vi "VISA Init --GPS--.vi"(2 "Error In":errorcluster, 3 "VISA resource name In":refnum<visa-resource-name>) -> (0 "Error Out":errorcluster, 1 "VISA resource name Out":refnum<visa-resource-name>)   [LabVIEW 2015]
uses:
  <vilib>/Instr/_visa.llb/VISA Configure Serial Port (Instr).vi
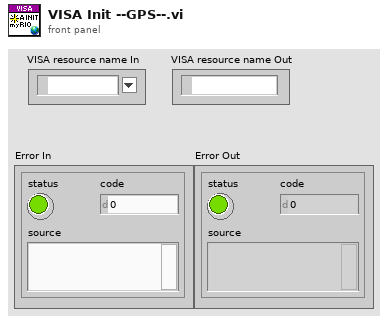
[diagram p1: front panel]
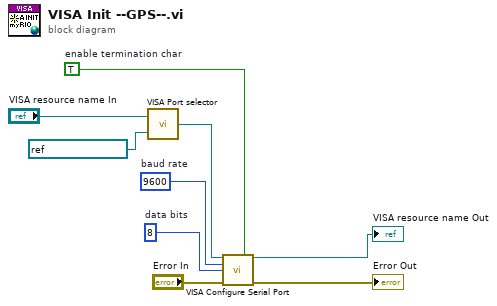
[diagram p0: block diagram]
diagram:
  w7 = TRUE  # enable termination char
  w8 = u16 8  # data bits
  w9 = u32 9600  # baud rate
  n1 = call "VISA Port selector.vi"("Defualt"=refnum<visa-resource-name> "ASRL1::INSTR" ("GPS"), "I/P"="VISA resource name In") -> ("O/P"=w6:refnum<visa-resource-name>)
  n2 = call-poly "VISA Configure Serial Port"("VISA resource name"=w6, "Enable Termination\nChar (T)"=w7, "baud rate (9600)"=w9, "data bits (8)"=w8, "error in (no error)"="Error In") -> ("VISA resource name out"=→"VISA resource name Out":refnum<visa-resource-name>, "error out"=→"Error Out":errorcluster)  [unwired: 9 in]
